vi "swabian_retrieve_histogram.vi"(8 "error in (no error)":errorcluster, 11 "swabian_local_data":T1={"events"={"update_status"=refnum, "update_chart"=refnum, "update_xy"=refnum, "send_channel_data"=refnum}, "stop_q"=refnum, "tagger_reference"=refnum, "connect_button"=refnum, "counter_reference"=refnum, "tagger_stream_reference"=refnum, "log_reference"=refnum, "current_log_offset"=0, "tt20_buffer_q"=refnum, "stream_to_file_button"=refnum, "num_records"=0, "connected?"=FALSE, "plots"=refnum, "histogram_bin_edges"=[], "histogrammer"=refnum, "plot_lifetimes"=refnum, "xy_graph"=refnum, "Reference\nChannel"=enum."ch0"}) -> (0 "error out":errorcluster, 2 "stop":bool, 3 "swabian_local_data 2":T1={"events"={"update_status"=refnum, "update_chart"=refnum, "update_xy"=refnum, "send_channel_data"=refnum}, "stop_q"=refnum, "tagger_reference"=refnum, "connect_button"=refnum, "counter_reference"=refnum, "tagger_stream_reference"=refnum, "log_reference"=refnum, "current_log_offset"=0, "tt20_buffer_q"=refnum, "stream_to_file_button"=refnum, "num_records"=0, "connected?"=FALSE, "plots"=refnum, "histogram_bin_edges"=[], "histogrammer"=refnum, "plot_lifetimes"=refnum, "xy_graph"=refnum, "Reference\nChannel"=enum."ch0"})   [LabVIEW 2015]
uses:
  swabian_local_data_tdef.ctl
  swabian_events_tdef.ctl
  update_chart_tdef.ctl
  channel_data_tdef.ctl
  C:/Users/bspoka/Dropbox (MIT)/Swabian/lib/TTCSharp32.dll
  lib/TTCSharp32.dll
  swabian_buffer_tdef.ctl
  reference_checkbox_tdef.ctl
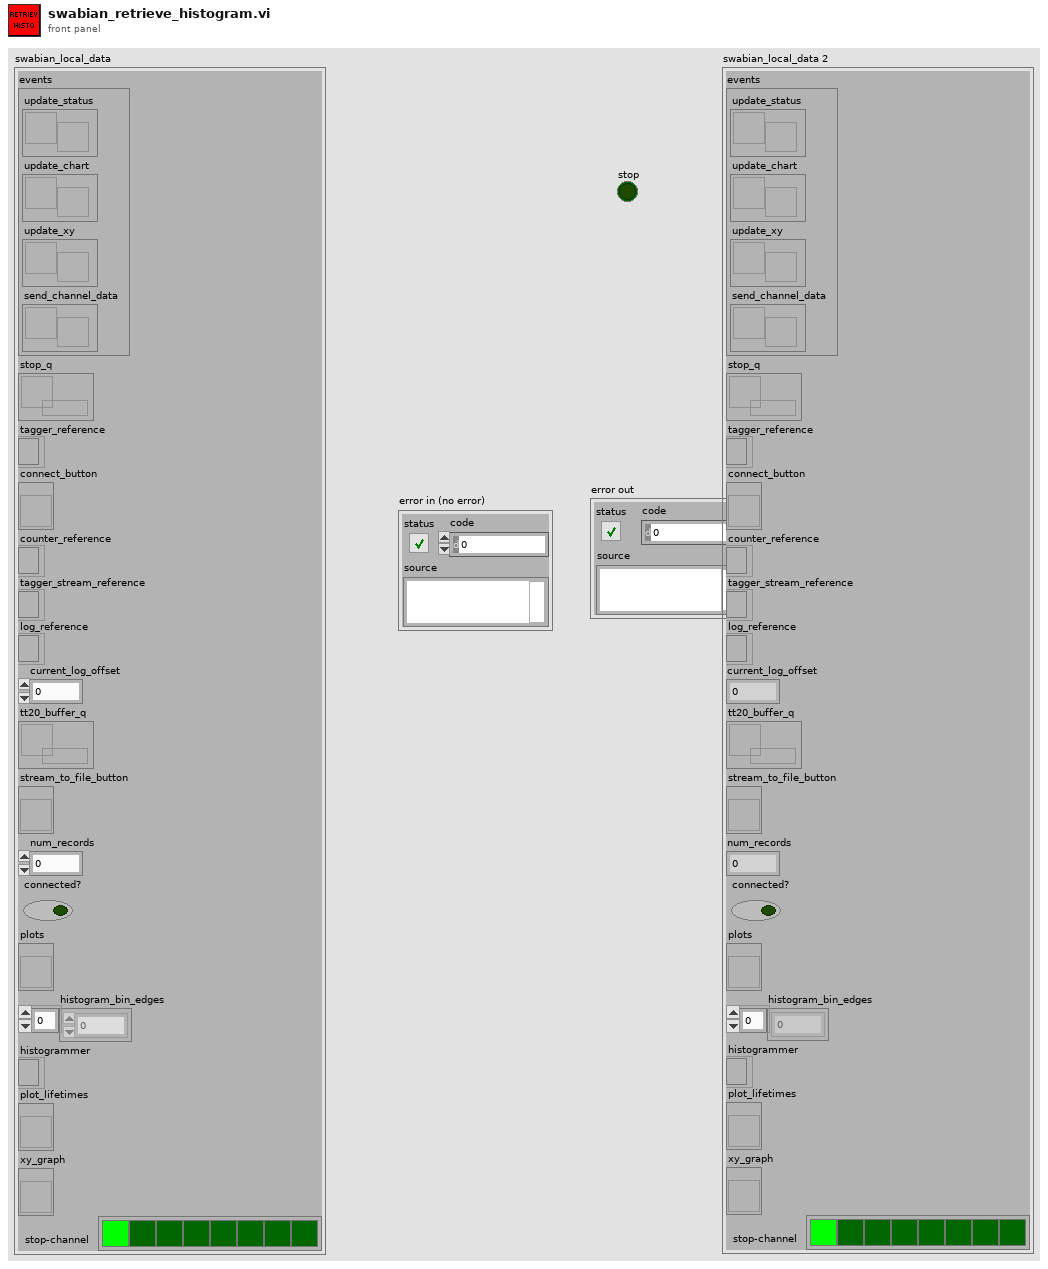
[diagram p1: front panel]
types:
  T1 = typedef "swabian_local_data_tdef.ctl" = cluster{"events":T2, "stop_q":refnum<queue>, "tagger_reference":refnum<k24>, "connect_button":refnum<vi>, "counter_reference":refnum<k24>, "tagger_stream_reference":refnum<k24>, "log_reference":refnum<file>, "current_log_offset":i64, "tt20_buffer_q":refnum<queue>, "stream_to_file_button":refnum<vi>, "num_records":u64, "connected?":bool, "plots":refnum<vi>, "histogram_bin_edges":i64[], "histogrammer":refnum<k24>, "plot_lifetimes":refnum<vi>, "xy_graph":refnum<vi>, "Reference\nChannel":T3}
  T2 = typedef "swabian_events_tdef.ctl" = cluster{"update_status":refnum<user-event>, "update_chart":refnum<user-event>, "update_xy":refnum<user-event>, "send_channel_data":refnum<user-event>}
  T3 = typedef "reference_checkbox_tdef.ctl" = enum32{"No Selection", "ch0", "ch1", "ch2", "ch3", "ch4", "ch5", "ch6", "ch7"}
  T4 = typedef "channel_data_tdef.ctl" = cluster{"data":cluster{dbl[], dbl[]}, "channel":u8}
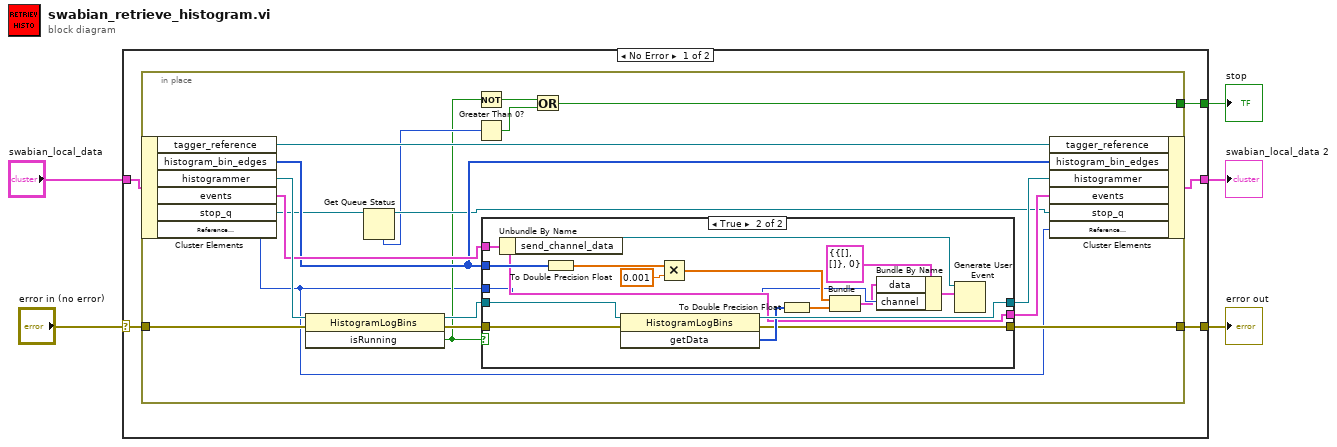
[diagram p0: block diagram]
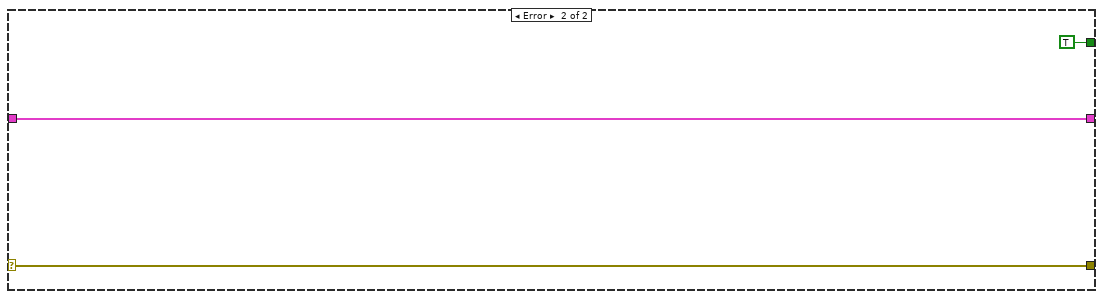
[diagram p3: hidden frame]
diagram:
  n1 = case shown="No Error" "error in (no error)" {
    selector: "error in (no error)" -> [w9 w49]
    tunnel: "swabian_local_data" -> [w10 w50]
    tunnel: [w7 w49] -> w5
    tunnel: [w8 w50] -> w4
    tunnel: [w6 TRUE ("isRunning")] -> w1
    frame No Error {
      n2 = in-place {
        in-place-border: w9 -> [w26]
        in-place-border: [w23] -> w7
        in-place-border: [w13] -> w6
        n3 = in-place-cluster #1(w10) -> ("tagger_reference"=w28:refnum<k24>, "histogram_bin_edges"=w22:i64[], "histogrammer"=w27:refnum<k24>, "events"=w25:T2, "stop_q"=w18:refnum<queue>, "Reference\nChannel"=w11:T3)
        n4 = invoke class="HistogramLogBins" method="isRunning"(reference=w27, error in=w26) -> (reference out=w20:refnum<k24>, error out=w19:errorcluster, "isRunning"=w12:bool)  [unwired: 1 in]
        n5 = Get Queue Status(queue=w18) -> (queue out=w17:refnum<queue>, # elements in queue=w16:i32)  [unwired: 2 in, 6 out]
        n6 = Not(x=w12) -> (.not. x?=w15:bool)
        n7 = Greater Than 0?(x=w16) -> (x > 0?=w14:bool)
        n8 = case shown="True" w12 {
          tunnel: w25 -> [w31 w37]
          tunnel: [w31 w37] -> w24
          tunnel: [w29 w36] -> w23
          tunnel: w22 -> [_ w47]
          tunnel: [w30 w46] -> w21
          tunnel: w20 -> [w30 w45]
          tunnel: w19 -> [w29 w44]
          tunnel: w11 -> [_ w35]
          frame False {
          }
          frame True {
            n9 = Unbundle By Name(w37) -> ("send_channel_data"=w38:refnum<user-event>)
            n10 = To Double Precision Float(number=w47) -> (double precision float=w40:dbl[])
            n11 = invoke class="HistogramLogBins" method="getData"(reference=w45, error in=w44) -> (reference out=w46:refnum<k24>, error out=w36:errorcluster, "getData"=w43:u64[])  [unwired: 1 in]
            n12 = Multiply(x=w40, y=0.001) -> (x*y=w39:dbl[])
            n13 = To Double Precision Float(number=w43) -> (double precision float=w42:dbl[])
            n14 = Bundle(w39, w42) -> (w33:cluster{dbl[], dbl[]})  [unwired: 1 in]
            n15 = Bundle By Name(cluster=T4 {"data"={[], []}, "channel"=0} ("event data"), "data"=w33, "channel"=w35) -> (w32:T4)
            n16 = Generate User Event(user event=w38, event data cluster=w32) -> ()  [unwired: 2 in, 2 out]
          }
        }
        n17 = Or(x=w15, y=w14) -> (x .or. y?=w13:bool)
        n18 = in-place-cluster #1("tagger_reference"=w28, "histogram_bin_edges"=w22, "histogrammer"=w21, "events"=w24, "stop_q"=w17, "Reference\nChannel"=w11) -> (w8:T1)
      }
    }
    frame Error {
    }
  }
  "swabian_local_data 2" <- w4
  "error out" <- w5
  "stop" <- w1
